vi "uPublisher SimplePublish.vi"(8 "error in (no error)":errorcluster, 9 "Payload":refnum<class "uData.lvclass">, 10 "Topic":string, 11 "uClient_Publisher in":refnum<class "uClient_Publisher.lvclass">) -> (0 "error out":errorcluster, 3 "uClient_Publisher out":refnum<class "uClient_Publisher.lvclass">)   [LabVIEW 2021, in "uFramework.lvlib" / "uClient_Publisher.lvclass"]
doc: "Simplified non-optimized method to Publish a simple event to the broker.\nFor Full control over the event uMsg, use the 'Publish' method instead."
uses:
  uClient_Publisher.lvclass
  uClient_Publisher.lvclass/uClient_Publisher.ctl
  uMsg/uMsg.lvclass
  Bin/uData.lvlibp/uData.lvclass
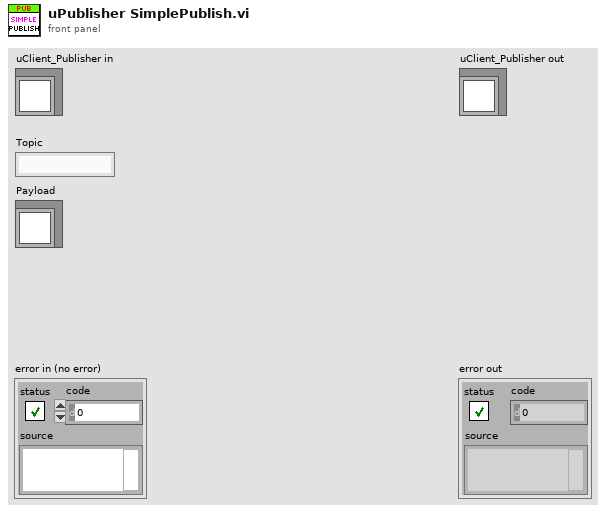
[diagram p1: front panel]
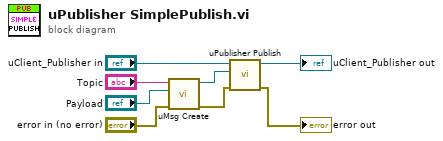
[diagram p0: block diagram]
diagram:
  n1 = call "uMsg Create.vi"("error in (no error)"="error in (no error)", "Payload"="Payload", "CMD"="Topic") -> ("error out"=w2:errorcluster, "uMsg out"=w1:refnum<class "uMsg.lvclass">)  [unwired: 7 in]
  n2 = call "uPublisher Publish.vi"("error in (no error)"=w2, "uMsg"=w1, "uClient_Publisher in"="uClient_Publisher in") -> ("error out"=→"error out":errorcluster, "uClient_Publisher out"=→"uClient_Publisher out":refnum<class "uClient_Publisher.lvclass">)  [unwired: 7 in]
